vi "initWithTimeStamp.vi"(8 "error in (no error)":errorcluster, 9 "timeStamp":string, 10 "computer name":string) -> (0 "error out":errorcluster, 3 "FileNeologist out":refnum<class "FileNeologist.lvclass">)   [LabVIEW 2009, in "Tools.lvlib" / "Filing.lvlib" / "FileNeologist.lvclass"]
doc: "FileNeologist Initialise.\n\nThe File Neologist is responsible for creating new files, and naming/renaming files."
uses:
  FileNeologist.lvclass
  FileNeologist.lvclass/FileNeologist.ctl
  FileSystem/FileSystem.lvclass
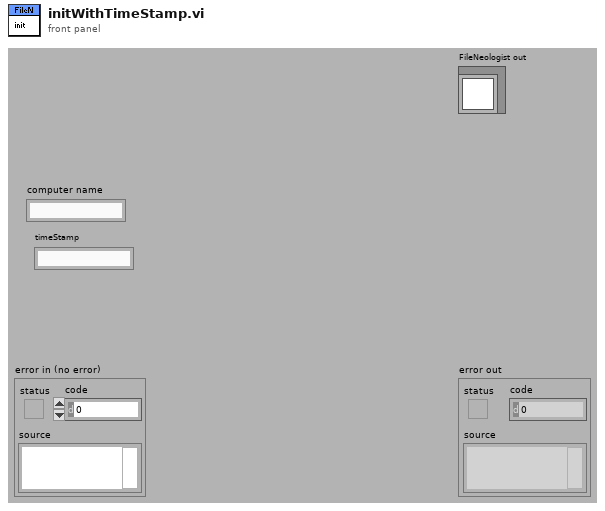
[diagram p1: front panel]
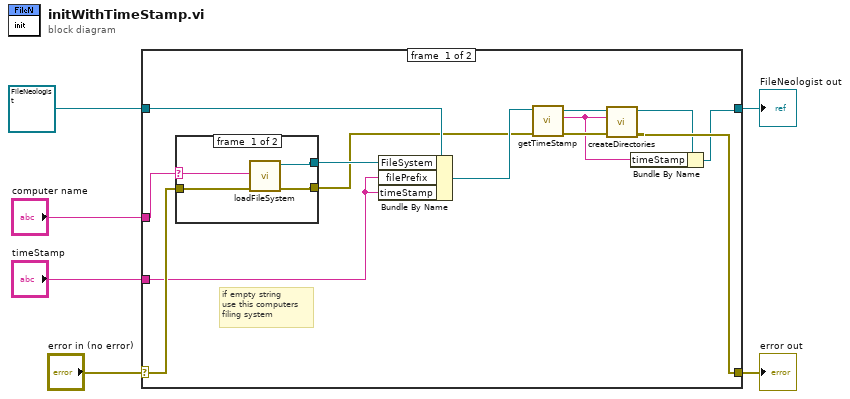
[diagram p0: block diagram]
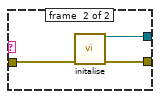
[diagram p2: hidden frame]
diagram:
  n1 = case shown="No Error" "error in (no error)" {
    selector: "error in (no error)" -> [w19 w28]
    tunnel: [w14 w28] -> w5
    tunnel: [w11 w27] -> w4
    tunnel: refnum<class "FileNeologist.lvclass"> refnum ("Tools.lvlib:Filing.lvlib:FileNeologist.lvclass") -> [w9 w27]
    tunnel: "computer name" -> [w10 _]
    tunnel: "timeStamp" -> [w7 _]
    frame #0 {
      # "if empty string\nuse this computers\nfiling system"
      n2 = case shown="\"\"" w10 {
        selector: w10 -> [w23 _]
        tunnel: w19 -> [w20 w26]
        tunnel: [w22 w25] -> w18
        tunnel: [w21 w24] -> w8
        frame #0 {
          n3 = call "loadFileSystem.vi"("error in (no error)"=w20, "computer name"=w23) -> ("error out"=w21:errorcluster, "FileSystem out"=w22:refnum<class "FileSystem.lvclass">)  [unwired: 8 in]
        }
        frame #1 {
          n4 = call "initalise.vi"("error in (no error)"=w26) -> ("error out"=w24:errorcluster, "FileSystem out"=w25:refnum<class "FileSystem.lvclass">)  [unwired: 9 in]
        }
      }
      n5 = Bundle By Name(cluster=w9, "FileSystem"=w18, "filePrefix"=w7, "timeStamp"=w7) -> (w17:refnum<class "FileNeologist.lvclass">)
      n6 = call "getTimeStamp.vi"("error in (no error)"=w8, "FileNeologist in"=w17) -> ("error out"=w15:errorcluster, "TimeStamp"=w13:string, "FileNeologist out"=w16:refnum<class "FileNeologist.lvclass">)  [unwired: 7 in]
      n7 = call "createDirectories.vi"("error in (no error)"=w15, "TimeStamp"=w13, "FileNeologist in"=w16) -> ("error out"=w14:errorcluster, "FileNeologist out"=w12:refnum<class "FileNeologist.lvclass">)  [unwired: 7 in]
      n8 = Bundle By Name(cluster=w12, "timeStamp"=w13) -> (w11:refnum<class "FileNeologist.lvclass">)
    }
    frame #1 {
    }
  }
  "error out" <- w5
  "FileNeologist out" <- w4
